vi "CameraTesting4.vi"() -> ()   [LabVIEW 2019]
doc: "The myRIO Project template acquires acceleration data from the onboard accelerometer and displays the changes of acceleration values in a waveform chart."
uses:
  <vilib>/myRIO/Express VI/Onboard IO/Encoder/Encoder Express VI.xnode
  <vilib>/myRIO/Common/Instrument Driver Framework/myRIO v1.0/Encoder/typedefs/Encoder Count Direction Enum.ctl
  <vilib>/myRIO/Instrument Drivers/Onboard IO/Encoder/typedefs/Encoder Reference.ctl
  <vilib>/myRIO/Instrument Drivers/Onboard IO/Encoder/Encoder.lvlib
  <vilib>/myRIO/Common/Instrument Driver Framework/myRIO v1.0/Encoder/typedefs/Encoder Channels Enum.ctl
  <vilib>/myRIO/Common/Instrument Driver Framework/Utilities/typedefs/myRIO Generic Hardware Reference.ctl
  <vilib>/myRIO/Common/Instrument Driver Framework/Utilities/typedefs/myRIO v1.0 Reference.ctl
  <vilib>/myRIO/Common/Instrument Driver Framework/Utilities/typedefs/Generic FPGA Reference.ctl
  <vilib>/myRIO/Common/Instrument Driver Framework/Utilities/typedefs/Hardware Version Enum.ctl
  <vilib>/myRIO/Common/Instrument Driver Framework/myRIO v1.0/Encoder/typedefs/Encoder Signal Mode.ctl
  <vilib>/myRIO/Instrument Drivers/Onboard IO/Encoder/vis/Read.vi
  <vilib>/myRIO/Instrument Drivers/Onboard IO/Encoder/vis/myRIO Encoder Open.xnode
  <vilib>/userdefined/High Color/nirio_resource_hc.ctl
  <vilib>/myRIO/Common/Instrument Driver Framework/myRIO v1.0/Encoder/typedefs/Encoder Configuration v1.0.ctl
  <vilib>/myRIO/Common/Instrument Driver Framework/myRIO v1.0/Encoder/vis/myRIO v1.1 Open Encoder.vi
  <vilib>/myRIO/Common/Instrument Driver Framework/myRIO v1.0/Encoder/vis/myRIO v1.0 Configure Encoder.vi
  <vilib>/myRIO/Common/Instrument Driver Framework/Utilities/vis/Is FPGA Ref Available.vi
  <vilib>/myRIO/Express VI/Onboard IO/PWM/PWM Express VI.xnode
  <vilib>/myRIO/Instrument Drivers/Onboard IO/PWM/vis/Set Duty Cycle and Frequency.vi
  <vilib>/myRIO/Instrument Drivers/Onboard IO/PWM/PWM.lvlib
  <vilib>/myRIO/Instrument Drivers/Onboard IO/PWM/typedefs/PWM Configuration.ctl
  <vilib>/myRIO/Common/Instrument Driver Framework/myRIO v1.0/PWM/typedefs/PWM Channels Enum.ctl
  <vilib>/myRIO/Instrument Drivers/Onboard IO/PWM/typedefs/PWM Reference.ctl
  <vilib>/myRIO/Instrument Drivers/Onboard IO/PWM/vis/myRIO PWM Open.xnode
  <vilib>/myRIO/Common/Instrument Driver Framework/myRIO v1.0/PWM/vis/myRIO v1.1 Open PWM.vi
panel:
  out "Pause":i32
  out "WaitTime":dbl=1000.0
  out "FrameRate":i32=30
  out "Stop":bool
  out "VidTS":dbl[][](array[numeric])
  out "GoVid":i32=1
  out "VidFrameClock":i32
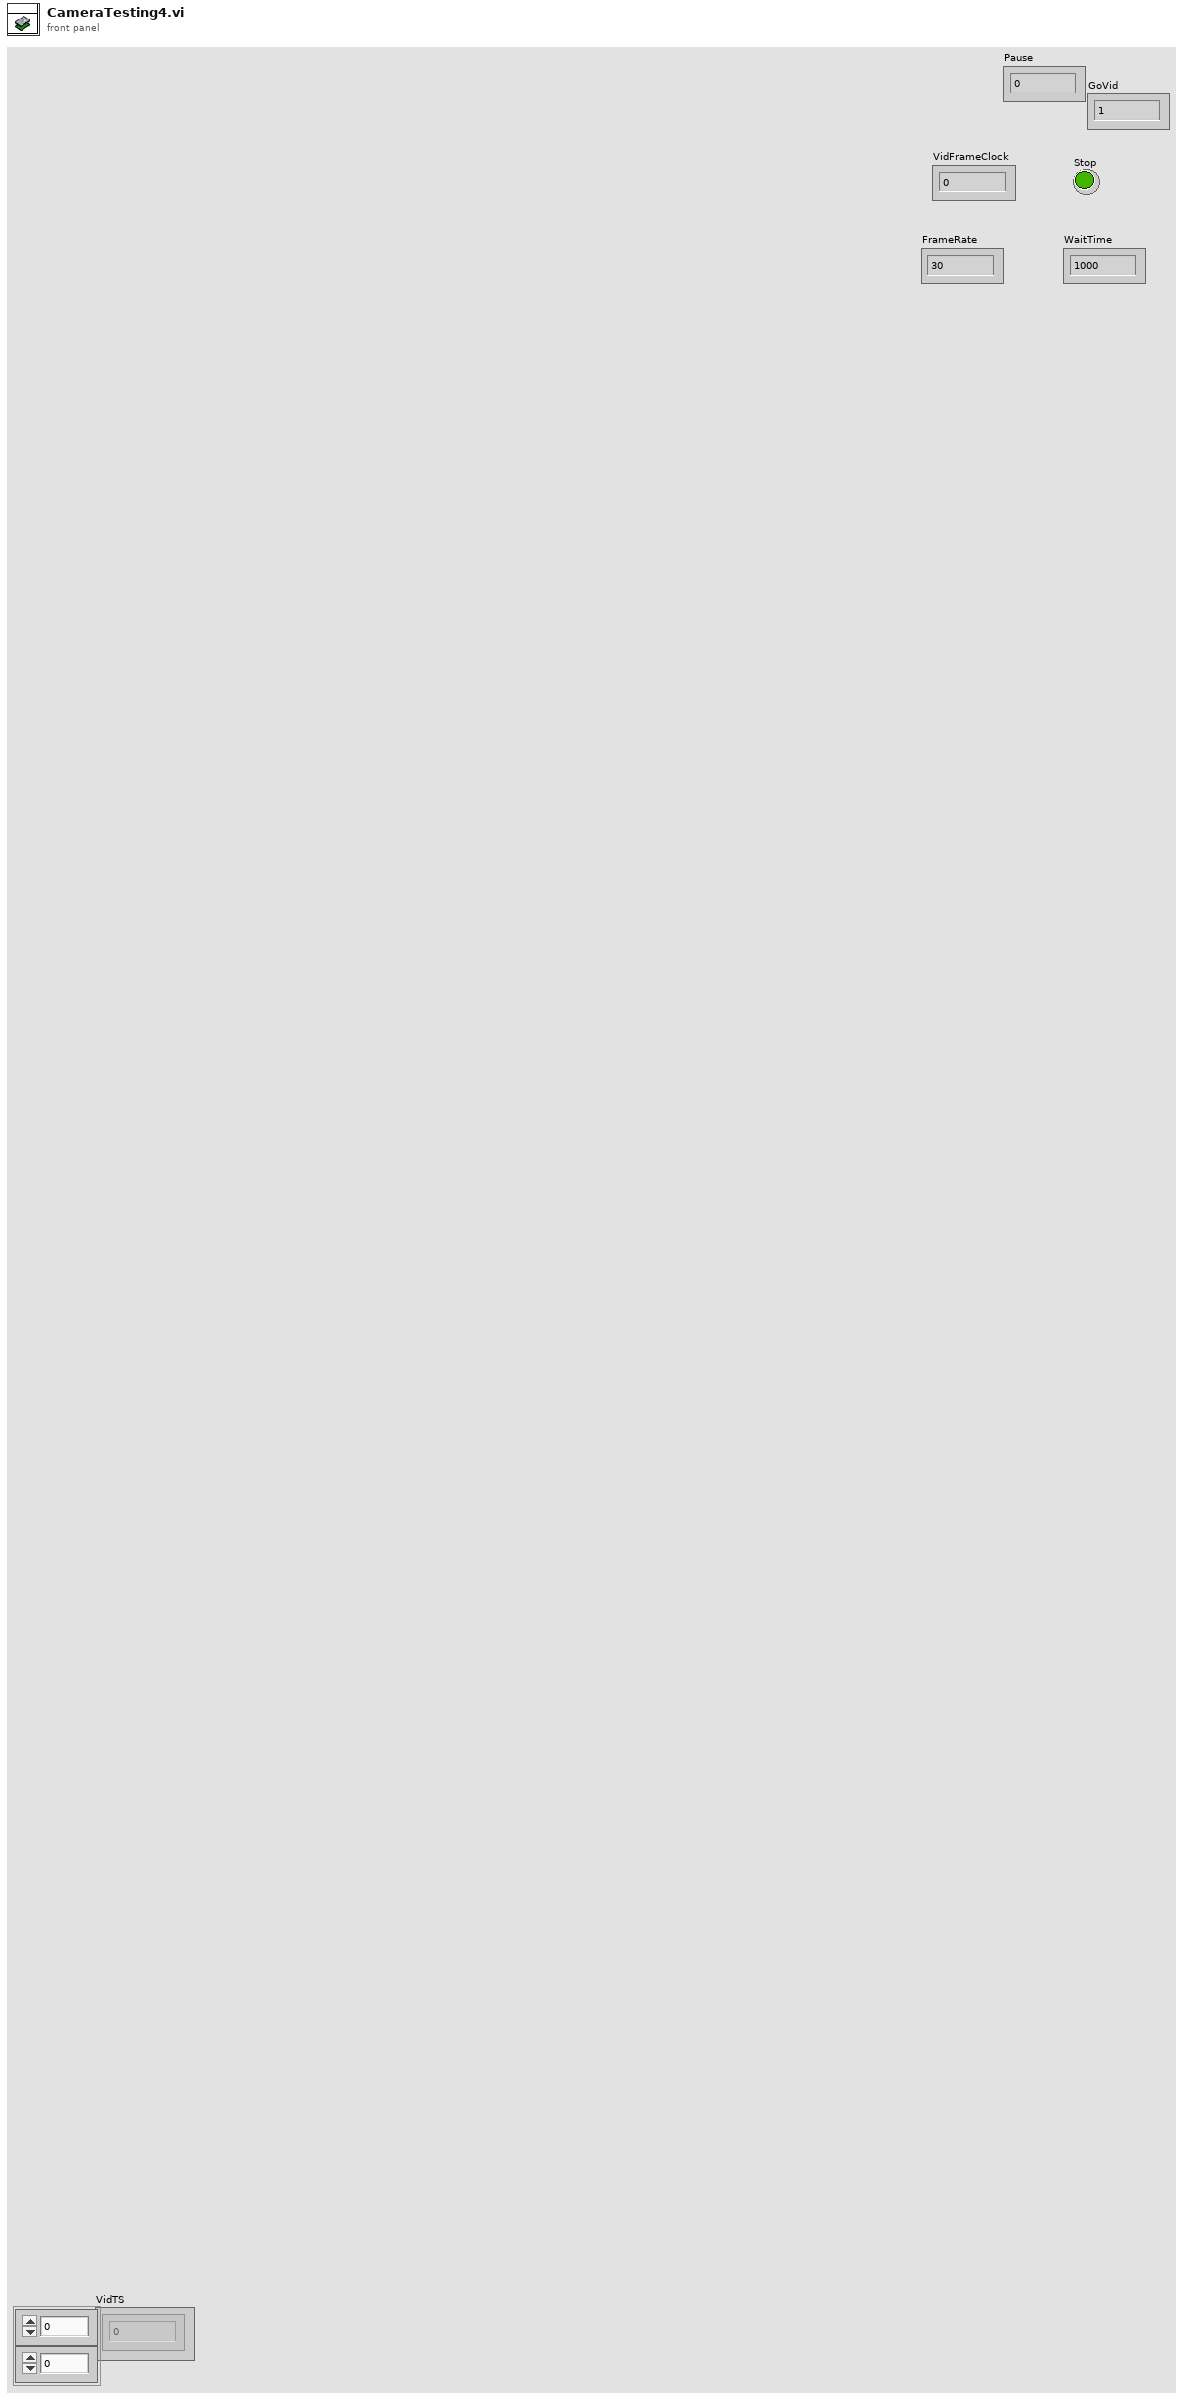
[diagram p1: front panel]
types:
  T1 = typedef "Encoder.lvlib/Encoder Reference.ctl" = cluster{"myRIO Reference":T2, "Encoder Channels Enum":T6}
  T2 = typedef "myRIO Generic Hardware Reference.ctl" = cluster{"myRIO Model":T3, "myRIO Hardware Reference":T4}
  T3 = typedef "Hardware Version Enum.ctl" = enum16{"Unknown", "myRIO-1900", "myRIO-1950", "roboRIO", "NI ELVIS RIO CM", "ELVIS III"}
  T4 = typedef "myRIO v1.0 Reference.ctl" = cluster{"Generic FPGA Reference":T5, "Allow multiple opens":bool}
  T5 = typedef "Generic FPGA Reference.ctl" = refnum<k20>
  T6 = typedef "Encoder Channels Enum.ctl" = enum16{"Not Connected", "C/ENC0", "C/ENC1", "A/ENC", "A/ENC0", "A/ENC1", "A/ENC2", "A/ENC3", "A/ENC4", "A/ENC5", "A/ENC6", "A/ENC7", "A/ENC8", "A/ENC9", "B/ENC", "B/ENC0", "B/ENC1", "B/ENC2", "B/ENC3", "B/ENC4", "B/ENC5", "B/ENC6", "B/ENC7", "B/ENC8", "B/ENC9", "DIO/ENC0", "DIO/ENC1", "DIO/ENC2", "DIO/ENC3", "DIO/ENC4"}
  T7 = typedef "Encoder Signal Mode.ctl" = enum16{"Quadrature phase signal", "Step and direction signal"}
  T8 = typedef "nirio_resource_hc.ctl" = tag
  T9 = typedef "NI_Matrix.lvlib/RealMatrix.ctl" = dbl[][]
  T10 = typedef "PWM.lvlib/PWM Reference.ctl" = cluster{"myRIO Reference":T2, "PWM Channels Enum":T11, "PWM Configuration":T12}
  T11 = typedef "PWM Channels Enum.ctl" = enum16{"Not Connected", "C/PWM0", "C/PWM1", "A/PWM0", "A/PWM1", "A/PWM2", "A/PWM3", "A/PWM4", "A/PWM5", "A/PWM6", "A/PWM7", "A/PWM8", "A/PWM9", "A/PWM10", "A/PWM11", "A/PWM12", "A/PWM13", "A/PWM14", "A/PWM15", "A/PWM16", "A/PWM17", "A/PWM18", "A/PWM19", "B/PWM0", "B/PWM1", "B/PWM2", "B/PWM3", "B/PWM4", "B/PWM5", "B/PWM6", "B/PWM7", "B/PWM8", "B/PWM9", "B/PWM10", "B/PWM11", "B/PWM12", "B/PWM13", "B/PWM14", "B/PWM15", "B/PWM16", "B/PWM17", "B/PWM18", "B/PWM19", "PWM/PWM0", "PWM/PWM1", "PWM/PWM2", "PWM/PWM3", "PWM/PWM4", "PWM/PWM5", "PWM/PWM6", "PWM/PWM7", "PWM/PWM8", "PWM/PWM9"}
  T12 = typedef "PWM.lvlib/PWM Configuration.ctl" = cluster{"Frequency":dbl, "Duty Cycle":dbl}
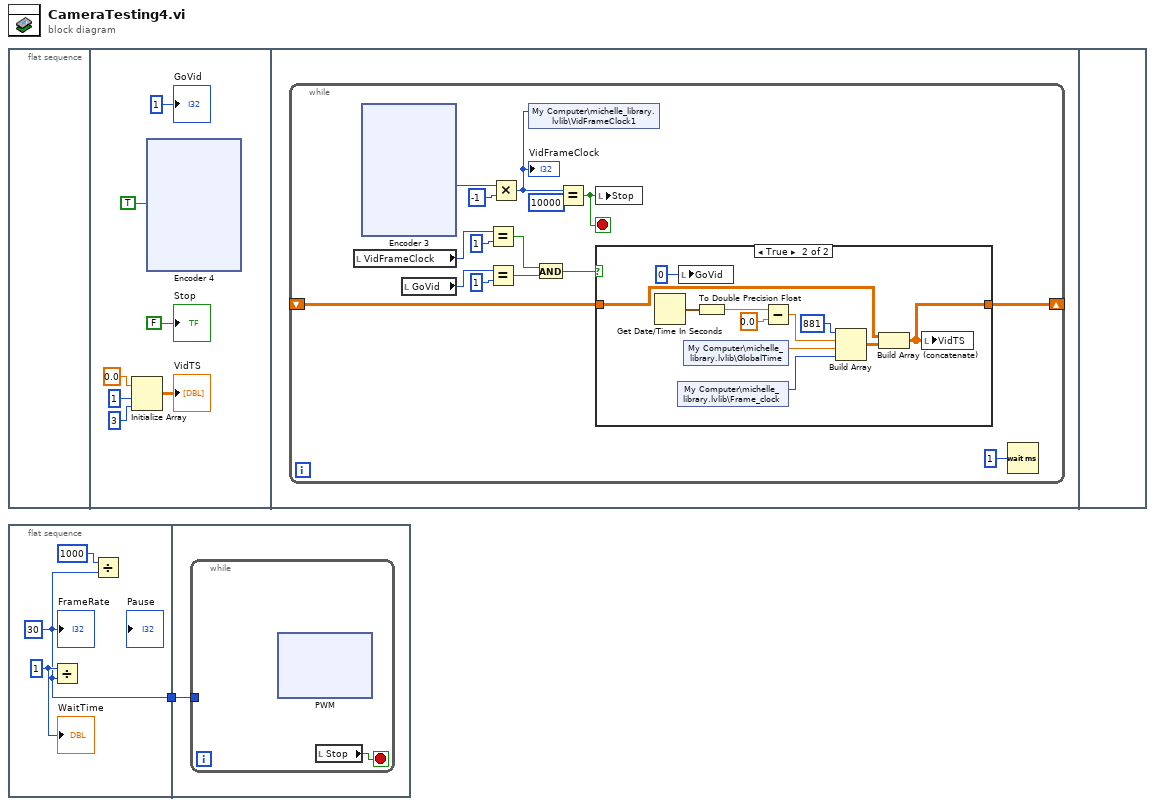
[diagram p0: block diagram]
diagram:
  n1 = flat-sequence {
    frame #0 {
    }
    frame #1 {
      n2 = Initialize Array(0.0, 1, 3) -> (→"VidTS":dbl[][])
      n3 = xnode "Encoder 4"("Reset Counter"=TRUE) -> ()  [unwired: 1 in, 4 out]
      "GoVid" <- 1
      "Stop" <- FALSE
    }
    frame #2 {
      n4 = while {
        shift-right: [w61] -> _
        shift-left: _ -> [w62]
        stop <- w66 stop-if-true
        n5 = local read "VidFrameClock"() -> (w60:i32)
        n6 = xnode "Encoder 3"() -> ("Counter Value"=w68:i32)  [unwired: 2 in, 3 out]
        n7 = local read "GoVid"() -> (w56:i32)
        n8 = Equal?(x=w60, y=1) -> (x = y?=w59:bool)
        n9 = Equal?(x=w56, y=1) -> (x = y?=w55:bool)
        n10 = Multiply(x=w68, y=-1) -> (x*y=w65:i32)
        "VidFrameClock" <- w65
        n11 = shared-variable "My Computer\\michelle_library.lvlib\\VidFrameClock1"(w65) -> ()  [unwired: 1 in, 1 out]
        n12 = And(x=w59, y=w55) -> (x .and. y?=w58:bool)
        n13 = Equal?(x=w65, y=10000) -> (x = y?=w66:bool)
        n14 = local write "Stop"(w66) -> ()
        n15 = case shown="True" w58 {
          tunnel: w62 -> [w70 w74]
          tunnel: [w70 w73] -> w61
          frame False {
          }
          frame True {
            n16 = Get Date/Time In Seconds() -> (seconds since 1Jan1904=w81:timestamp)
            n17 = shared-variable "My Computer\\michelle_library.lvlib\\Frame_clock"() -> (w78:u32)  [unwired: 1 in, 1 out]
            n18 = local write "GoVid"(0) -> ()
            n19 = shared-variable "My Computer\\michelle_library.lvlib\\GlobalTime"() -> (w77:dbl)  [unwired: 1 in, 1 out]
            n20 = To Double Precision Float(number=w81) -> (double precision float=w80:dbl)
            n21 = Subtract(x=w80, y=0.0) -> (x-y=w79:dbl)
            n22 = Build Array(881, w79, w77, w78) -> (w76:T9)
            n23 = Build Array (concatenate) ("Build Matrix")(w74, w76) -> (w73:T9)
            n24 = local write "VidTS"(w73) -> ()
          }
        }
        n25 = Wait (ms)(milliseconds to wait=u32 1) -> ()  [unwired: 1 out]
      }
    }
    frame #3 {
    }
  }
  n26 = flat-sequence {
    tunnel: [w128] -> w1
    tunnel: w1 -> [w131]
    frame #0 {
      w130 = 1
      w128 = 30
      n27 = Divide(x=w130, y=w128) -> ()  [unwired: 1 out]
      n28 = Divide(x=1000, y=w128) -> ()  [unwired: 1 out]
      "FrameRate" <- w128
      "WaitTime" <- w130
    }
    frame #1 {
      n29 = while {
        tunnel: w131 -> [_]
        stop <- w132 stop-if-true
        n30 = xnode "PWM"() -> ()  [unwired: 1 in, 1 out]
        n31 = local read "Stop"() -> (w132:bool)
      }
    }
  }
